vi "Ramp (G3)-Compute Max Level.vi"(0 "Ramp.Properties":T3, 9 "Level":T1, 11 "error in (no error)":errorcluster) -> (6 "Max Level":dbl, 10 "Level out":T1, 15 "error out":errorcluster)   [LabVIEW 2020]
uses:
  Ramp.Properties.ctl
  XControls/Level (G3)/Level Data.ctl
  XControls/Level (G3)/Level Units (G3).ctl
  PXI DAQ VIs/DAQ Engine VIs/PXI Globals.vi
  Utility VIs/Math VIs/Linear to dB (scalar).vi
  XControls/Level (G3)/Level (G3).xctl
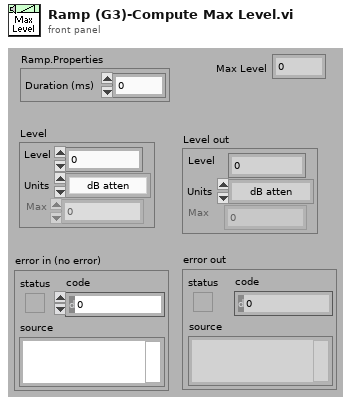
[diagram p1: front panel]
types:
  T1 = typedef "Level (G3).xctl/Level Data.ctl" = cluster{"Level":dbl, "Units":T2, "Max":dbl, "Data":cluster{"Multiplier":dbl, "Cal File":path, "Cal":cluster{"Freq (Hz)":dbl[], "Mag (dB SPL)":dbl[], "Phase (deg)":dbl[]}, "audiogram":path}}
  T2 = typedef "Level (G3).xctl/Level Units (G3).ctl" = enum16{"dB atten", "dB SPL", "dB re 1 Vrms", "dB V/Hz½", "mW", "dB HL", "Volts", "dB mW"}
  T3 = typedef "Ramp.Properties.ctl" = cluster{"Duration (ms)":dbl}
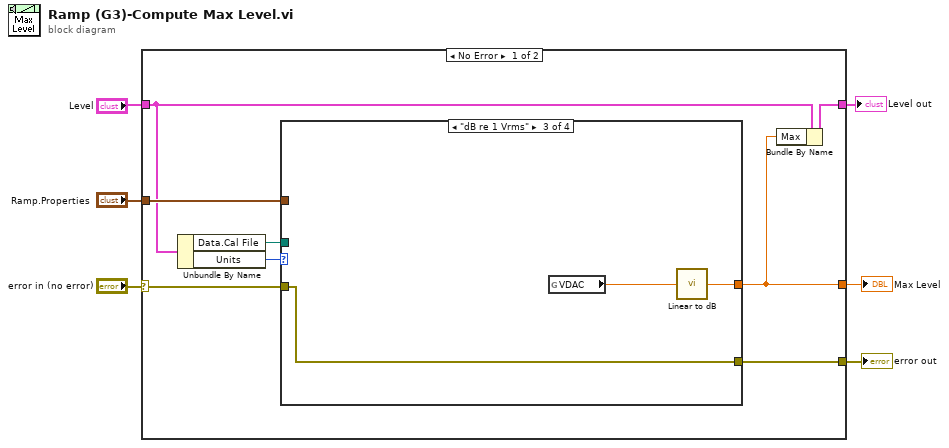
[diagram p0: block diagram]
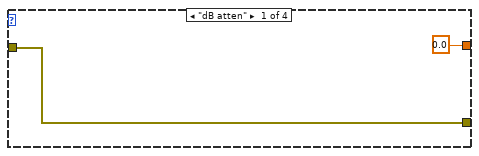
[diagram p2: hidden frame]
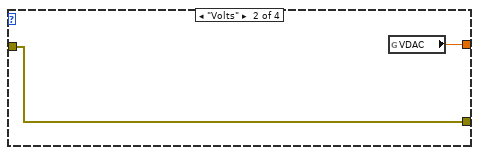
[diagram p3: hidden frame]
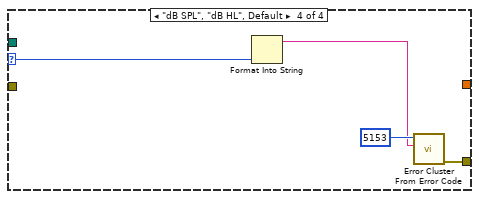
[diagram p4: hidden frame]
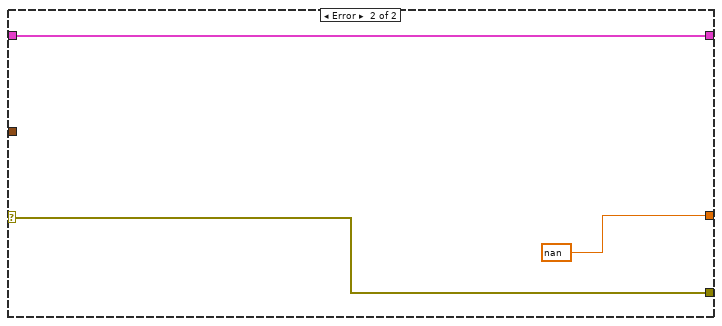
[diagram p5: hidden frame]
diagram:
  n1 = case shown="No Error" "error in (no error)" {
    selector: "error in (no error)" -> [w14 w28]
    tunnel: "Level" -> [w11 w26]
    tunnel: "Ramp.Properties" -> [w13 _]
    tunnel: [w12 w28] -> w5
    tunnel: [w10 nan ("Reference Level")] -> w2
    tunnel: [w9 w26] -> w1
    frame No Error {
      n2 = Unbundle By Name(w11) -> ("Data.Cal File"=w8:path, "Units"=w7:T2)
      n3 = case shown="\"dB re 1 Vrms\"" w7 {
        selector: w7 -> [_ _ _ w23]
        tunnel: w14 -> [w15 w18 w21 _]
        tunnel: w13 -> [_ _ _ _]
        tunnel: [0.0 ("Reference Level") w17 w19 _] -> w10
        tunnel: [w15 w18 w21 w25] -> w12
        tunnel: w8 -> [_ _ _ _]
        frame "dB atten" {
        }
        frame "Volts" {
          n4 = global read "PXI Globals.vi" "VDAC"() -> (w17:dbl)
        }
        frame "dB re 1 Vrms" {
          n5 = global read "PXI Globals.vi" "VDAC"() -> (w20:dbl)
          n6 = call-poly "Linear to dB.vi"("Linear"=w20) -> ("dB"=w19:dbl)
        }
        frame "dB SPL", "dB HL", Default {
          n7 = Format Into String(w23) -> (resulting string=w22:string)  [unwired: 3 in, 1 out]
          n8 = call <vilib>:"Error Cluster From Error Code.vi"("error message (\"\")"=w22, "error code (0)"=5153) -> ("error out"=w25:errorcluster)  [unwired: 7 in]
        }
      }
      n9 = Bundle By Name(cluster=w11, "Max"=w10) -> (w9:T1)
    }
    frame Error {
    }
  }
  "error out" <- w5
  "Max Level" <- w2
  "Level out" <- w1
